vi "Save As.vi"(8 "error in (no error)":errorcluster, 11 "path":path) -> (0 "error out":errorcluster, 2 "File Path":path, 3 "File Name":string)   [LabVIEW 2021]
panel:
  in  "Enter File Name":string
  in  "Cancel":bool
  in  "Save":bool
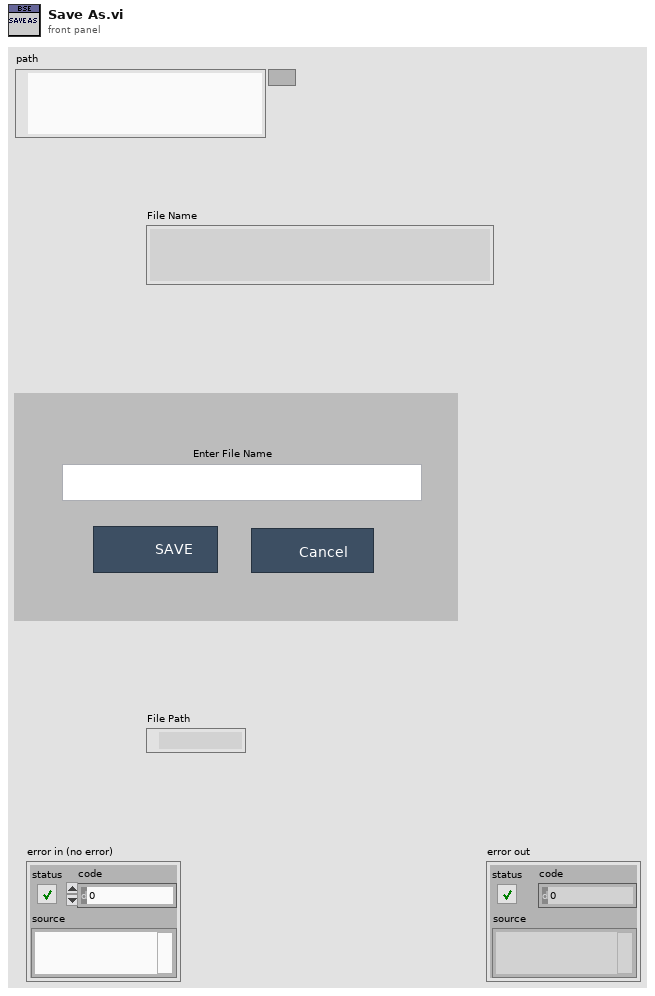
[diagram p1: front panel]
types:
  T1 = enum16{"open", "replace", "create", "open or create", "replace or create", "replace or create with confirmation"}
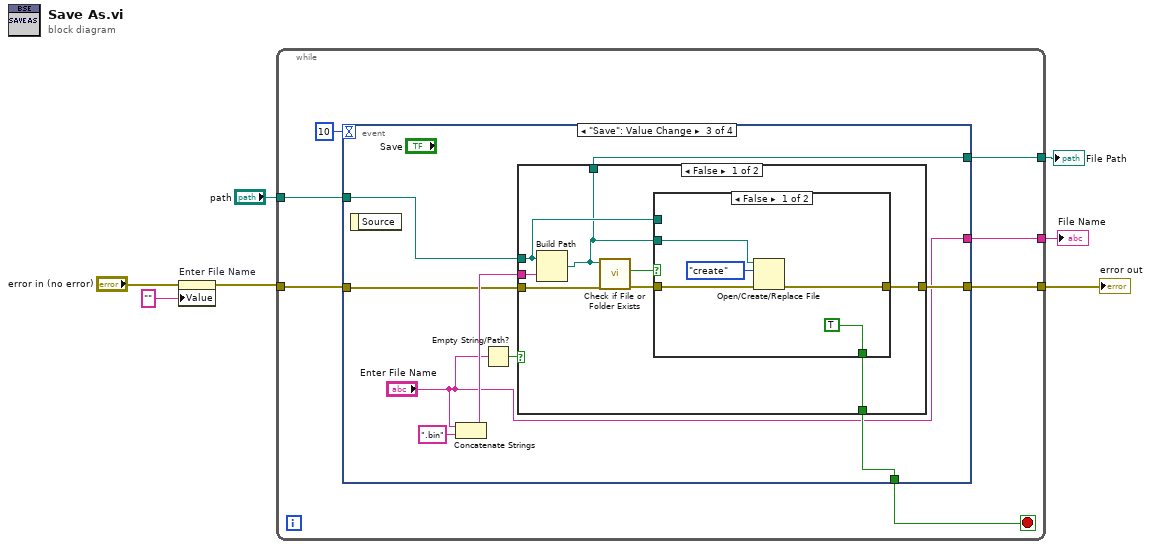
[diagram p0: block diagram]
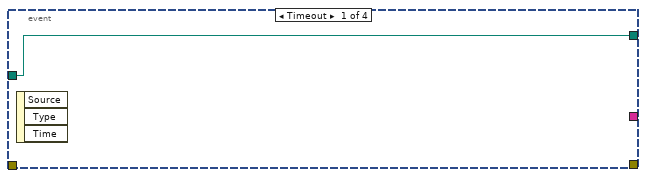
[diagram p2: hidden frame]
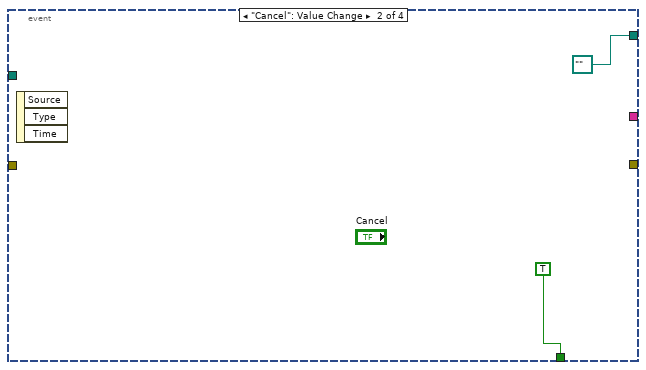
[diagram p3: hidden frame]
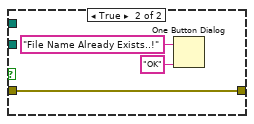
[diagram p4: hidden frame]
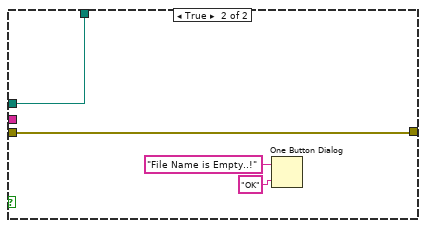
[diagram p5: hidden frame]
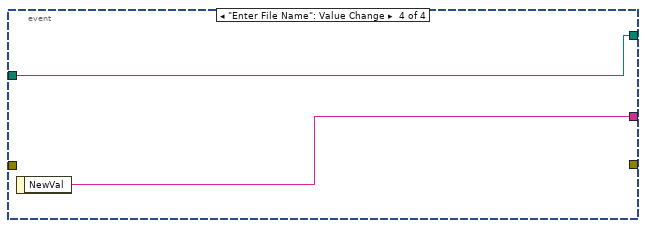
[diagram p6: hidden frame]
diagram:
  n1 = property on="Enter File Name" class="Str"(error in="error in (no error)", "Value"="" ("Enter File Name")) -> (error out=w3:errorcluster)  [unwired: 1 in, 1 out]
  n2 = while {
    tunnel: w3 -> [w9]
    tunnel: [w13] -> w7
    tunnel: "path" -> [w10]
    tunnel: [w11] -> w5
    tunnel: [w8] -> w4
    stop <- w12 stop-if-true
    n3 = event shown="[2] \"Save\": Value Change" {
      selector: _ -> [_ _ _ _]
      dyn-events: _ -> [_ _ _ _]
      timeout: 10 -> [_ _ _ _]
      tunnel: [_ _ w26 _] -> w13
      tunnel: [_ TRUE ("Cancel") w21 _] -> w12
      tunnel: [_ _ "Enter File Name" w48] -> w11
      tunnel: w10 -> [w15 _ w22 w47]
      tunnel: w9 -> [_ _ w23 _]
      tunnel: [w15 path "" ("path") w20 w47] -> w8
      event Timeout {
        n4 = event-data() -> ()  [unwired: 1 in, 3 out]
      }
      event "Cancel": Value Change {
        n5 = event-data() -> ()  [unwired: 1 in, 3 out]
      }
      event "Save": Value Change {
        n6 = event-data() -> ()  [unwired: 1 in, 1 out]
        n7 = Concatenate Strings("Enter File Name", ".bin" ("string")) -> (w25:string)
        n8 = Empty String/Path?(string/path="Enter File Name") -> (empty?=w19:bool)
        n9 = case shown="False" w19 {
          tunnel: [w32 w45] -> w26
          tunnel: w25 -> [w31 _]
          tunnel: w23 -> [w30 w45]
          tunnel: w22 -> [w29 w46]
          tunnel: [w28 _] -> w21
          tunnel: [w27 w46] -> w20
          frame False {
            n10 = Build Path(base path=w29, name or relative path=w31) -> (appended path=w27:path)
            n11 = call <vilib>:"Check if File or Folder Exists.vi"("error in (no error)"=w30, "path"=w27) -> ("error out"=w33:errorcluster, "file or folder exists?"=w34:bool)  [unwired: 7 in, 1 out]
            n12 = case shown="False" w34 {
              tunnel: w33 -> [w39 w40]
              tunnel: [w38 w40] -> w32
              tunnel: w29 -> [_ _]
              tunnel: w27 -> [w37 _]
              tunnel: [TRUE ("Cancel") _] -> w28
              frame False {
                n13 = Open/Create/Replace File(file path (use dialog)=w37, error in=w39, operation (0:open)=T1."create") -> (error out=w38:errorcluster)  [unwired: 3 in, 2 out]
              }
              frame True {
                n14 = One Button Dialog(message="File Name Already Exists..!", button name ("OK")="OK") -> ()  [unwired: 1 out]
              }
            }
          }
          frame True {
            n15 = One Button Dialog(message="File Name is Empty..!", button name ("OK")="OK") -> ()  [unwired: 1 out]
          }
        }
      }
      event "Enter File Name": Value Change {
        n16 = event-data() -> ("NewVal"=w48:string)  [unwired: 1 in]
      }
    }
  }
  "error out" <- w7
  "File Name" <- w5
  "File Path" <- w4
